vi "Untitled 1.vi"() -> ()   [LabVIEW 2019]
panel:
  out "Resta de pares e impares":dbl
  out "Suma de impares de 500 a 1500":dbl
  in  "Stop buttom":bool
  out "Suma de pares de 100 a 2000":dbl
  # "Programa 1"
  # "Realizar un programa que sume todos los números pares de 100 hasta 2000 y a este\nresultado restarlo con la suma de los números impares del 500 hasta el 1500, muestre\nen pantalla el resultado."
  # "Hecho por Juan Andrés Bermúdez Gómez"
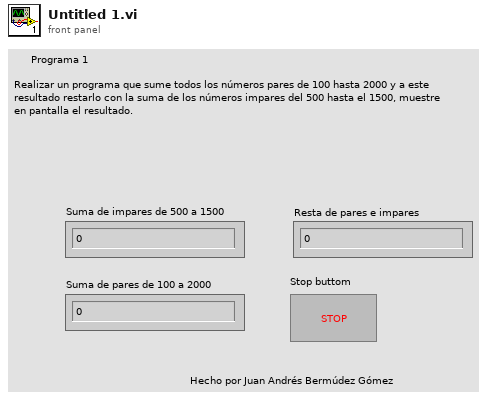
[diagram p1: front panel]
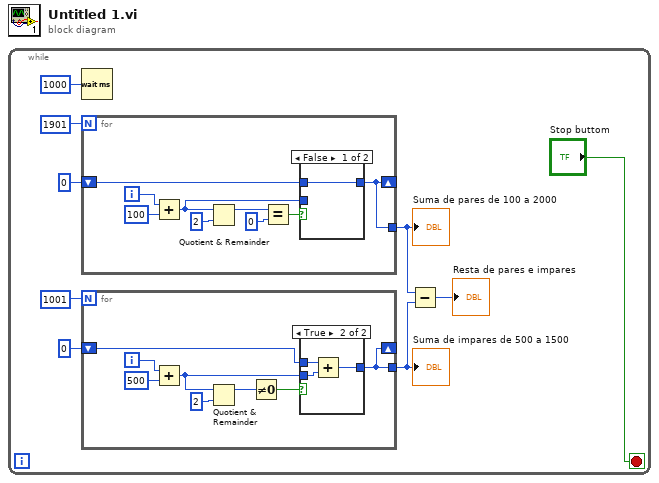
[diagram p0: block diagram]
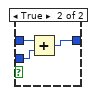
[diagram p3: hidden frame]
diagram:
  n1 = while {
    stop <- "Stop buttom" stop-if-true
    n2 = Wait (ms)(milliseconds to wait=u32 1000) -> ()  [unwired: 1 out]
    n3 = for {
      N: 1901 -> [_]
      shift-right: [w22] -> _
      shift-left: 0 -> [w28]
      tunnel: [w22] -> w3
      i -> [w30]
      n4 = Add(x=w30, y=100) -> (x+y=w25:i32)
      n5 = Quotient & Remainder(x=w25, y=2) -> (x-y*floor(x/y)=w24:i32)  [unwired: 1 out]
      n6 = Equal?(x=w24, y=0) -> (x = y?=w23:bool)
      n7 = case shown="False" w23 {
        tunnel: w28 -> [w31 w34]
        tunnel: [w31 w33] -> w22
        tunnel: w25 -> [_ w32]
        frame False {
        }
        frame True {
          n8 = Add(x=w34, y=w32) -> (x+y=w33:i32)
        }
      }
    }
    "Suma de pares de 100 a 2000" <- w3
    n9 = for {
      N: 1001 -> [_]
      shift-right: [w10] -> _
      shift-left: 0 -> [w12]
      tunnel: [w10] -> w2
      i -> [w17]
      n10 = Add(x=w17, y=500) -> (x+y=w11:i32)
      n11 = Quotient & Remainder(x=w11, y=2) -> (x-y*floor(x/y)=w14:i32)  [unwired: 1 out]
      n12 = Not Equal To 0?(x=w14) -> (x != 0?=w13:bool)
      n13 = case shown="True" w13 {
        tunnel: w12 -> [w18 w21]
        tunnel: w11 -> [_ w20]
        tunnel: [w18 w19] -> w10
        frame False {
        }
        frame True {
          n14 = Add(x=w21, y=w20) -> (x+y=w19:i32)
        }
      }
    }
    "Suma de impares de 500 a 1500" <- w2
    n15 = Subtract(x=w3, y=w2) -> (x-y=→"Resta de pares e impares":i32)
  }
